vi "Read String.vi"(8 "error in (no error)":errorcluster, 11 "class string child in":refnum<class "Child.lvclass">) -> (0 "error out":errorcluster, 2 "String":string, 3 "class string child out":refnum<class "Child.lvclass">)   [LabVIEW 2017, in "Child.lvclass"]
doc: "Gets the string data from Child.ctl"
uses:
  Child.lvclass
  Child.lvclass/Child.ctl
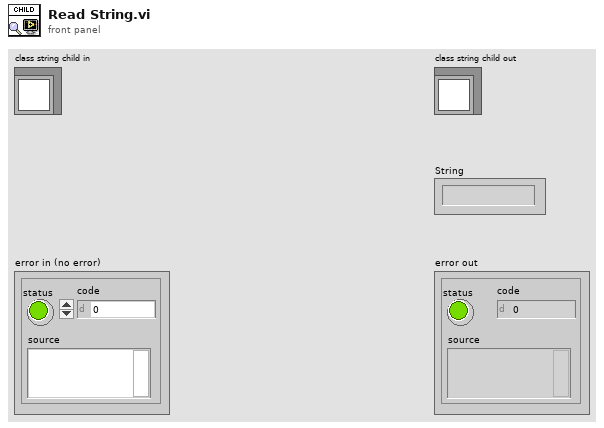
[diagram p1: front panel]
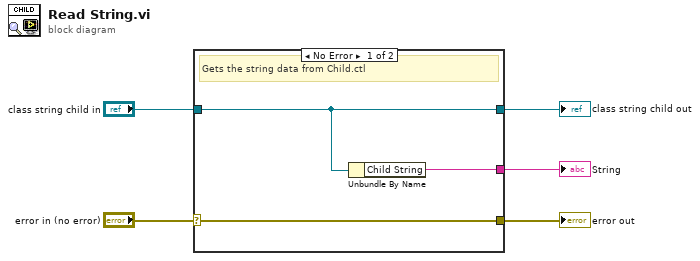
[diagram p0: block diagram]
diagram:
  n1 = case shown="No Error" "error in (no error)" {
    selector: "error in (no error)" -> [w8 w9]
    tunnel: [w8 w9] -> w4
    tunnel: [w6 w10] -> w2
    tunnel: "class string child in" -> [w6 w10]
    tunnel: [w7 _] -> w1
    frame No Error {
      # "Gets the string data from Child.ctl"
      n2 = Unbundle By Name(w6) -> ("Child String"=w7:string)
    }
    frame Error {
    }
  }
  "error out" <- w4
  "class string child out" <- w2
  "String" <- w1
